vi "Mode Read.vi"(4 "error in (no error)":errorcluster, 6 "Container State":T4, 7 "Display State In":T2) -> (0 "error out":errorcluster, 2 "Value":T1, 3 "Display State Out":T2)   [LabVIEW 2013]
uses:
  <vilib>/_xctls/Container State.ctl
  <vilib>/_xctls/XControlSupport.lvlib
  Typedefs/INTERNAL-DATA.ctl
  UI_TimeSelector.xctl
  State.ctl
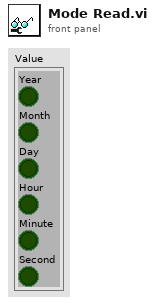
[diagram p1: front panel]
types:
  T1 = cluster{"Year":bool, "Month":bool, "Day":bool, "Hour":bool, "Minute":bool, "Second":bool}
  T2 = typedef "UI_TimeSelector.xctl/State.ctl" = cluster{"data":T3, "mode":cluster{"Year":bool, "Month":bool, "Day":bool, "Hour":bool, "Minute":bool, "Second":bool}}
  T3 = typedef "UI_TimeSelector.xctl/INTERNAL-DATA.ctl" = cluster{"year":string, "month":string, "day":string, "hour":string, "minute":string, "second":string}
  T4 = typedef "XControlSupport.lvlib/Container State.ctl" = cluster{"Indicator?":bool, "Run Mode?":bool, " Refnum":refnum<vi>}
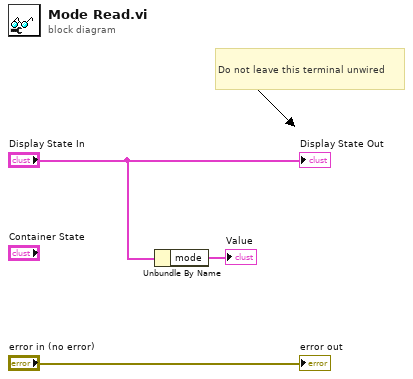
[diagram p0: block diagram]
diagram:
  # "Do not leave this terminal unwired"
  n1 = Unbundle By Name("Display State In") -> ("mode"=→"Value":T1)
  "error out" <- "error in (no error)"
  "Display State Out" <- "Display State In"
